vi "Update XY Graph With Multiple Plots in Real Time.vi"() -> ()   [LabVIEW 2009]
panel:
  in  "Number of Simulated Data Points":i32
  in  "Number of Plots":i32
  out "XY Graph":cluster{dbl[], dbl[]}[](graph)
  # "Source: https://decibel.ni.com/content/docs/DOC-32170"
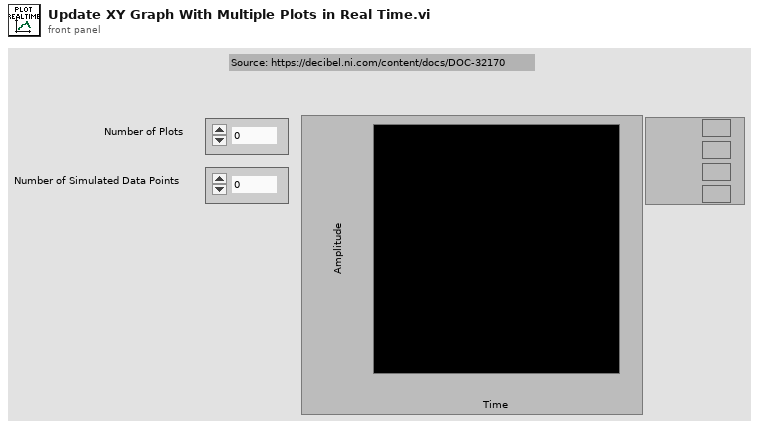
[diagram p1: front panel]
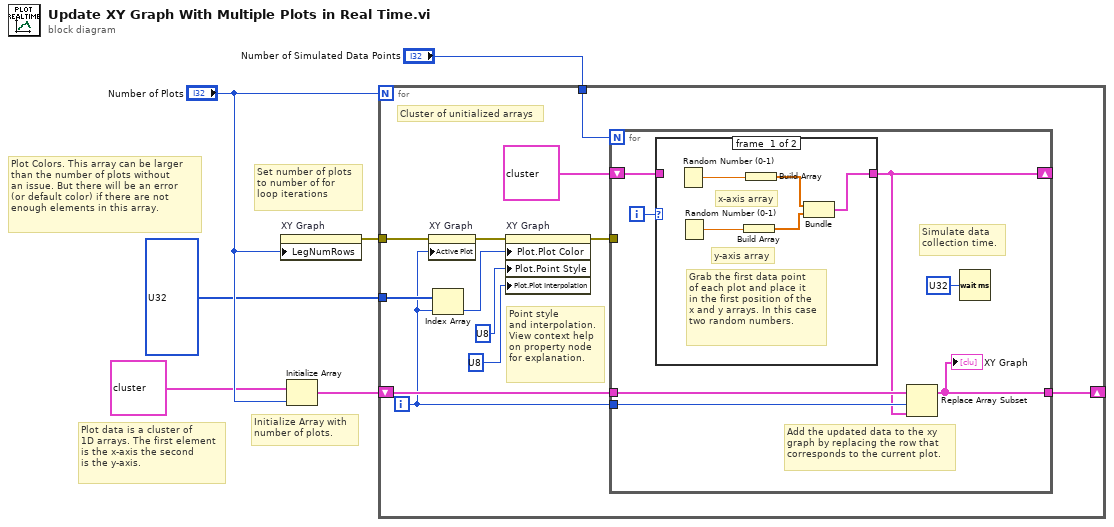
[diagram p0: block diagram]
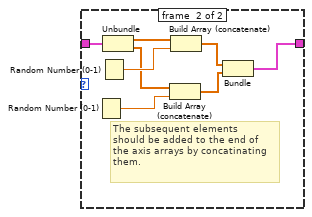
[diagram p2: hidden frame]
diagram:
  # "Plot Colors. This array can be larger \nthan the number of plots without\nan issue. But there will be an error\n(or default color) if there are not \nenough elements in this array."
  # "Plot data is a cluster of\n1D arrays. The first element\nis the x-axis the second\nis the y-axis."
  # "Set number of plots\nto number of for\nloop iterations"
  # "Initialize Array with \nnumber of plots."
  n1 = property on="XY Graph" class="XYGraph (strict)"("LegNumRows"="Number of Plots") -> (error out=w6:errorcluster)  [unwired: 2 in, 1 out]
  n2 = Initialize Array(cluster{dbl[], dbl[]} ?, "Number of Plots") -> (w4:cluster{dbl[], dbl[]}[])
  n3 = for {
    N: "Number of Plots" -> [_]
    tunnel: w6 -> [w14]
    shift-right: [w16] -> _
    shift-left: w4 -> [w18]
    tunnel: "Number of Simulated Data Points" -> [w15]
    tunnel: u32[] ? -> [w11]
    i -> [w10]
    # "Point style\nand interpolation.\nView context help\non property node\nfor explanation."
    # "Cluster of unitialized arrays"
    n4 = property on="XY Graph" class="XYGraph (strict)"(error in=w14, "Active Plot"=w10) -> (error out=w13:errorcluster)  [unwired: 1 in, 1 out]
    n5 = Index Array(array=w11, index=w10) -> (element=w9:u32)
    n6 = property on="XY Graph" class="XYGraph (strict)"(error in=w13, "Plot.Plot Color"=w9, "Plot.Point Style"=u8 ? ("Plot.Plot Interpolation"), "Plot.Plot Interpolation"=u8 ?) -> (error out=w8:errorcluster)  [unwired: 1 in, 1 out]
    n7 = for {
      N: w15 -> [_]
      tunnel: w18 -> [w23]
      shift-right: [w21] -> _
      shift-left: cluster{dbl[], dbl[]} ? -> [w24]
      tunnel: w10 -> [w22]
      tunnel: [w19] -> w16
      tunnel: w8 -> [_]
      i -> [w25]
      # "Add the updated data to the xy\ngraph by replacing the row that\ncorresponds to the current plot."
      # "Simulate data\ncollection time."
      n8 = case shown="1, Default" w25 {
        tunnel: [w28 w32] -> w21
        tunnel: w24 -> [_ w38]
        frame #0 {
          # "y-axis array"
          # "x-axis array"
          # "Grab the first data point\nof each plot and place it\nin the first position of the \nx and y arrays. In this case\ntwo random numbers."
          n9 = Random Number (0-1)() -> (number: 0 to 1=w27:dbl)
          n10 = Random Number (0-1)() -> (number: 0 to 1=w26:dbl)
          n11 = Build Array(w26) -> (w29:dbl[])
          n12 = Build Array(w27) -> (w30:dbl[])
          n13 = Bundle(w30, w29) -> (w28:cluster{dbl[], dbl[]})  [unwired: 1 in]
        }
        frame #1 {
          # "The subsequent elements\nshould be added to the end of\nthe axis arrays by concatinating\nthem."
          n14 = Random Number (0-1)() -> (number: 0 to 1=w35:dbl)
          n15 = Random Number (0-1)() -> (number: 0 to 1=w37:dbl)
          n16 = Unbundle(w38) -> (w36:dbl[], w31:dbl[])
          n17 = Build Array (concatenate)(w31, w35) -> (w33:dbl[])
          n18 = Build Array (concatenate)(w36, w37) -> (w34:dbl[])
          n19 = Bundle(w34, w33) -> (w32:cluster{dbl[], dbl[]})  [unwired: 1 in]
        }
      }
      n20 = Replace Array Subset(array=w23, new element=w21, index=w22) -> (w19:cluster{dbl[], dbl[]}[])
      "XY Graph" <- w19
      n21 = Wait (ms)(milliseconds to wait=u32 ?) -> ()  [unwired: 1 out]
    }
  }
